vi "Target Vector Shift.vi"(8 "Shift":i32, 11 "Input Vector":dbl[](array[numeric])) -> (3 "Output Vector":dbl[](array[numeric]))   [LabVIEW 2018, in "COBRA Iterative Learning Control Library.lvlib"]
uses:
  COBRA Iterative Learning Control Library.lvlib
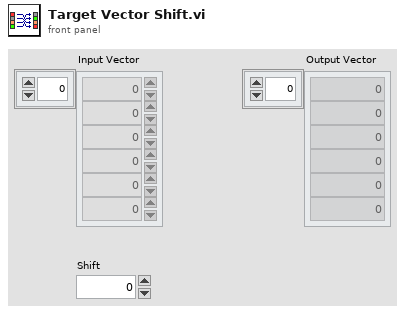
[diagram p1: front panel]
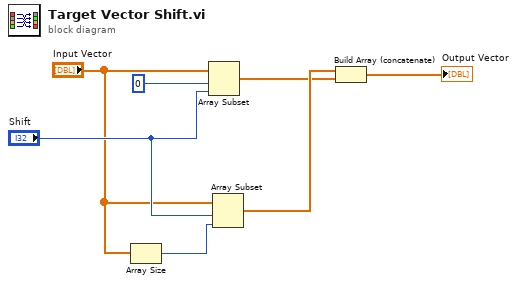
[diagram p0: block diagram]
diagram:
  n1 = Array Size(array="Input Vector") -> (size(s)=w4:i32)
  n2 = Array Subset "Array Subset"(array="Input Vector", index=0, length="Shift") -> (w2:dbl[])
  n3 = Array Subset "Array Subset"(array="Input Vector", index="Shift", length=w4) -> (w3:dbl[])
  n4 = Build Array (concatenate) "Build Array"(w3, w2) -> (→"Output Vector":dbl[])
